vi "Listbox Test.vi"() -> ()   [LabVIEW 2016]
panel:
  out "Focus Row":i32
  out "Time":u32
  in  "String":string
  out "size(s)":i32
  out "Selection Mode":i32
  out "Number of Rows":u32
  in  "Add Button":bool
  in  "stop":bool
  in  "Listbox":i32(listbox)
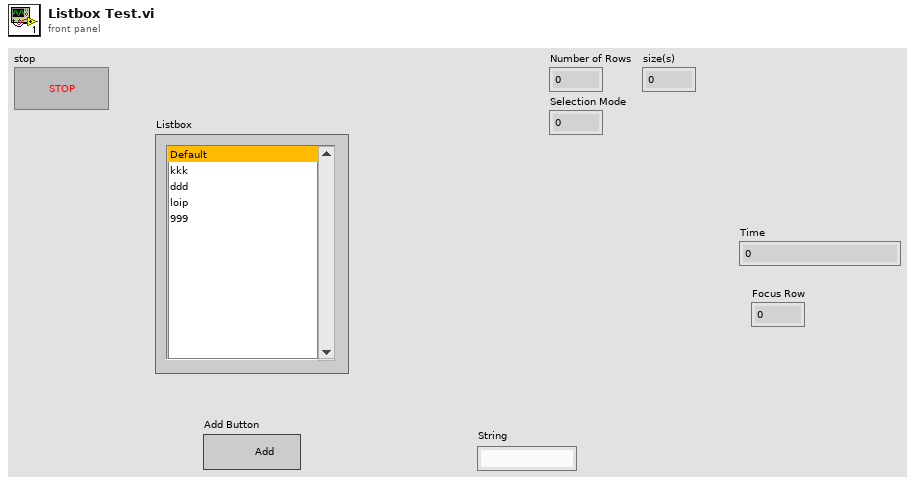
[diagram p1: front panel]
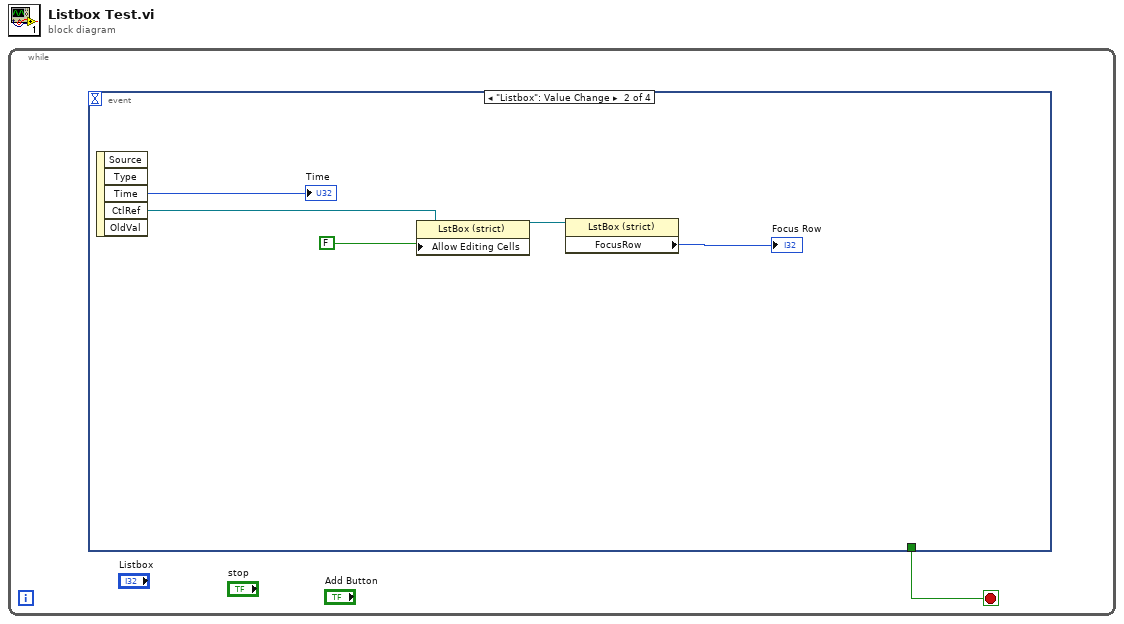
[diagram p0: block diagram]
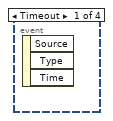
[diagram p2: hidden frame]
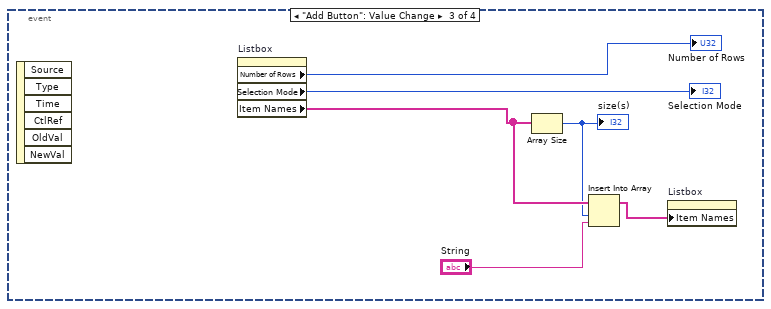
[diagram p3: hidden frame]
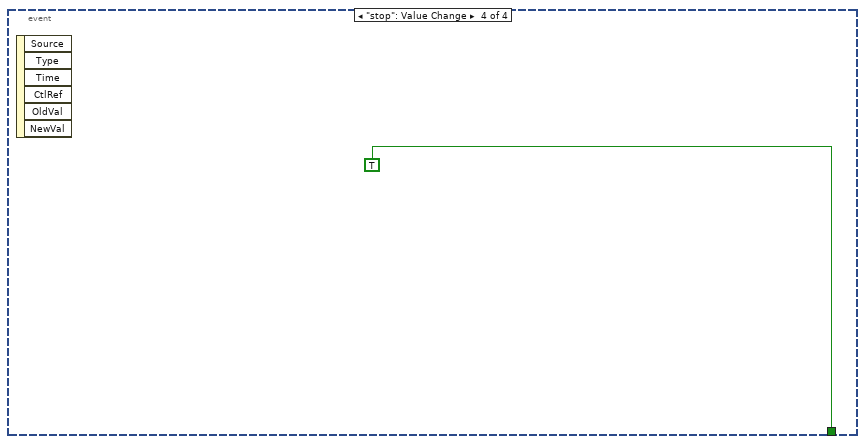
[diagram p4: hidden frame]
diagram:
  n1 = while {
    stop <- w1 stop-if-true
    n2 = event shown="[1] \"Listbox\": Value Change" {
      selector: _ -> [_ _ _ _]
      dyn-events: _ -> [_ _ _ _]
      timeout: _ -> [_ _ _ _]
      tunnel: [_ _ _ TRUE] -> w1
      event Timeout {
        n3 = event-data() -> ()  [unwired: 1 in, 3 out]
      }
      event "Listbox": Value Change {
        n4 = event-data() -> ("Time"=→"Time":u32, "CtlRef"=w5:refnum<vi>)  [unwired: 1 in, 3 out]
        n5 = property class="LstBox (strict)"(reference=w5, "Allow Editing Cells"=FALSE) -> (reference out=w3:refnum<vi>)  [unwired: 1 in, 1 out]
        n6 = property class="LstBox (strict)"(reference=w3) -> ("FocusRow"=→"Focus Row":i32)  [unwired: 1 in, 2 out]
      }
      event "Add Button": Value Change {
        n7 = event-data() -> ()  [unwired: 1 in, 6 out]
        n8 = property on="Listbox" class="LstBox (strict)"() -> ("Number of Rows"=→"Number of Rows":u32, "Selection Mode"=→"Selection Mode":i32, "Item Names"=w10:string[])  [unwired: 2 in, 2 out]
        n9 = Array Size(array=w10) -> (size(s)=w9:i32)
        "size(s)" <- w9
        n10 = Insert Into Array(array=w10, index=w9, new element="String") -> (w7:string[])
        n11 = property on="Listbox" class="LstBox (strict)"("Item Names"=w7) -> ()  [unwired: 2 in, 2 out]
      }
      event "stop": Value Change {
        n12 = event-data() -> ()  [unwired: 1 in, 6 out]
      }
    }
  }
